vi "Remove Request From Server.vi"(8 "error in":errorcluster, 10 "ReqIndex":i32, 11 "State Cluster":T1) -> (0 "error out":errorcluster)   [LabVIEW 2015]
uses:
  TypeDef/State Cluster.ctl
  LVClasses/Room/Room.lvclass
  LVClasses/Room/Room.lvclass/Room.ctl
  LVClasses/Room/Read Room Number.vi
  LVClasses/Room/Read RoomRequests.vi
  LVRestAPI/RoomRestApi.lvlib
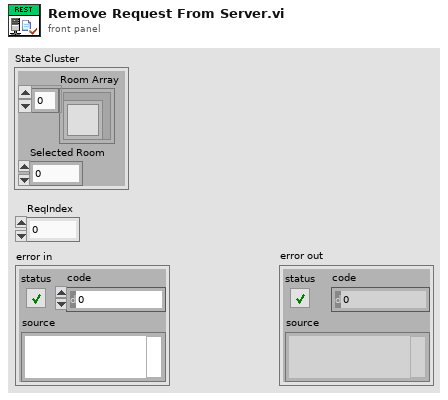
[diagram p1: front panel]
types:
  T1 = typedef "State Cluster.ctl" = cluster{"Room Array":refnum<class "Room.lvclass">[], "Selected Room":u32}
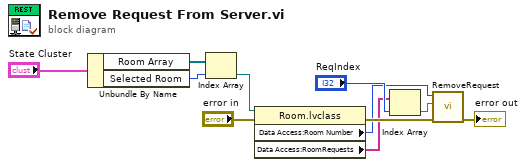
[diagram p0: block diagram]
diagram:
  n1 = Unbundle By Name("State Cluster") -> ("Room Array"=w9:refnum<class "Room.lvclass">[], "Selected Room"=w10:u32)
  n2 = Index Array(array=w9, index=w10) -> (element=w8:refnum<class "Room.lvclass">)
  n3 = property class="Room.lvclass"(reference=w8, error in="error in") -> (error out=w6:errorcluster, "Data Access:Room Number"=w1:i32, "Data Access:RoomRequests"=w2:string[])  [unwired: 1 out]
  n4 = Index Array(array=w2, index="ReqIndex") -> (element=w4:string)
  n5 = call "RemoveRequest.vi"("error in (no error)"=w6, "Request"=w4, "Room Number"=w1) -> ("error out"=→"error out":errorcluster)  [unwired: 7 in, 1 out]
